vi "Helium Test - Step 1.vi"(7 "Step":i32, 8 "error in":errorcluster, 9 "Test Results In":T9, 10 "Gas":T8, 11 "Test Configuration":T1) -> (0 "error out":errorcluster, 1 "Test Results Out":T9, 2 "Gas Out":T8 caption="Gas", 3 "Test Configuration Out":T1)   [LabVIEW 2015]
uses:
  CAN Communication/PAS/Typedefs/Session Handle.ctl
  CAN Communication/PAS/PAS.lvclass
  Controls/Test Results.ctl
  Controls/Step Result.ctl
  Controls/Test Configuration.ctl
  Controls/Vacuum Test.ctl
  Controls/Test Timing.ctl
  Controls/Vaccum Thresholds.ctl
  Controls/Helium Test.ctl
  Controls/Helium Thresholds.ctl
  Controls/Functional Test.ctl
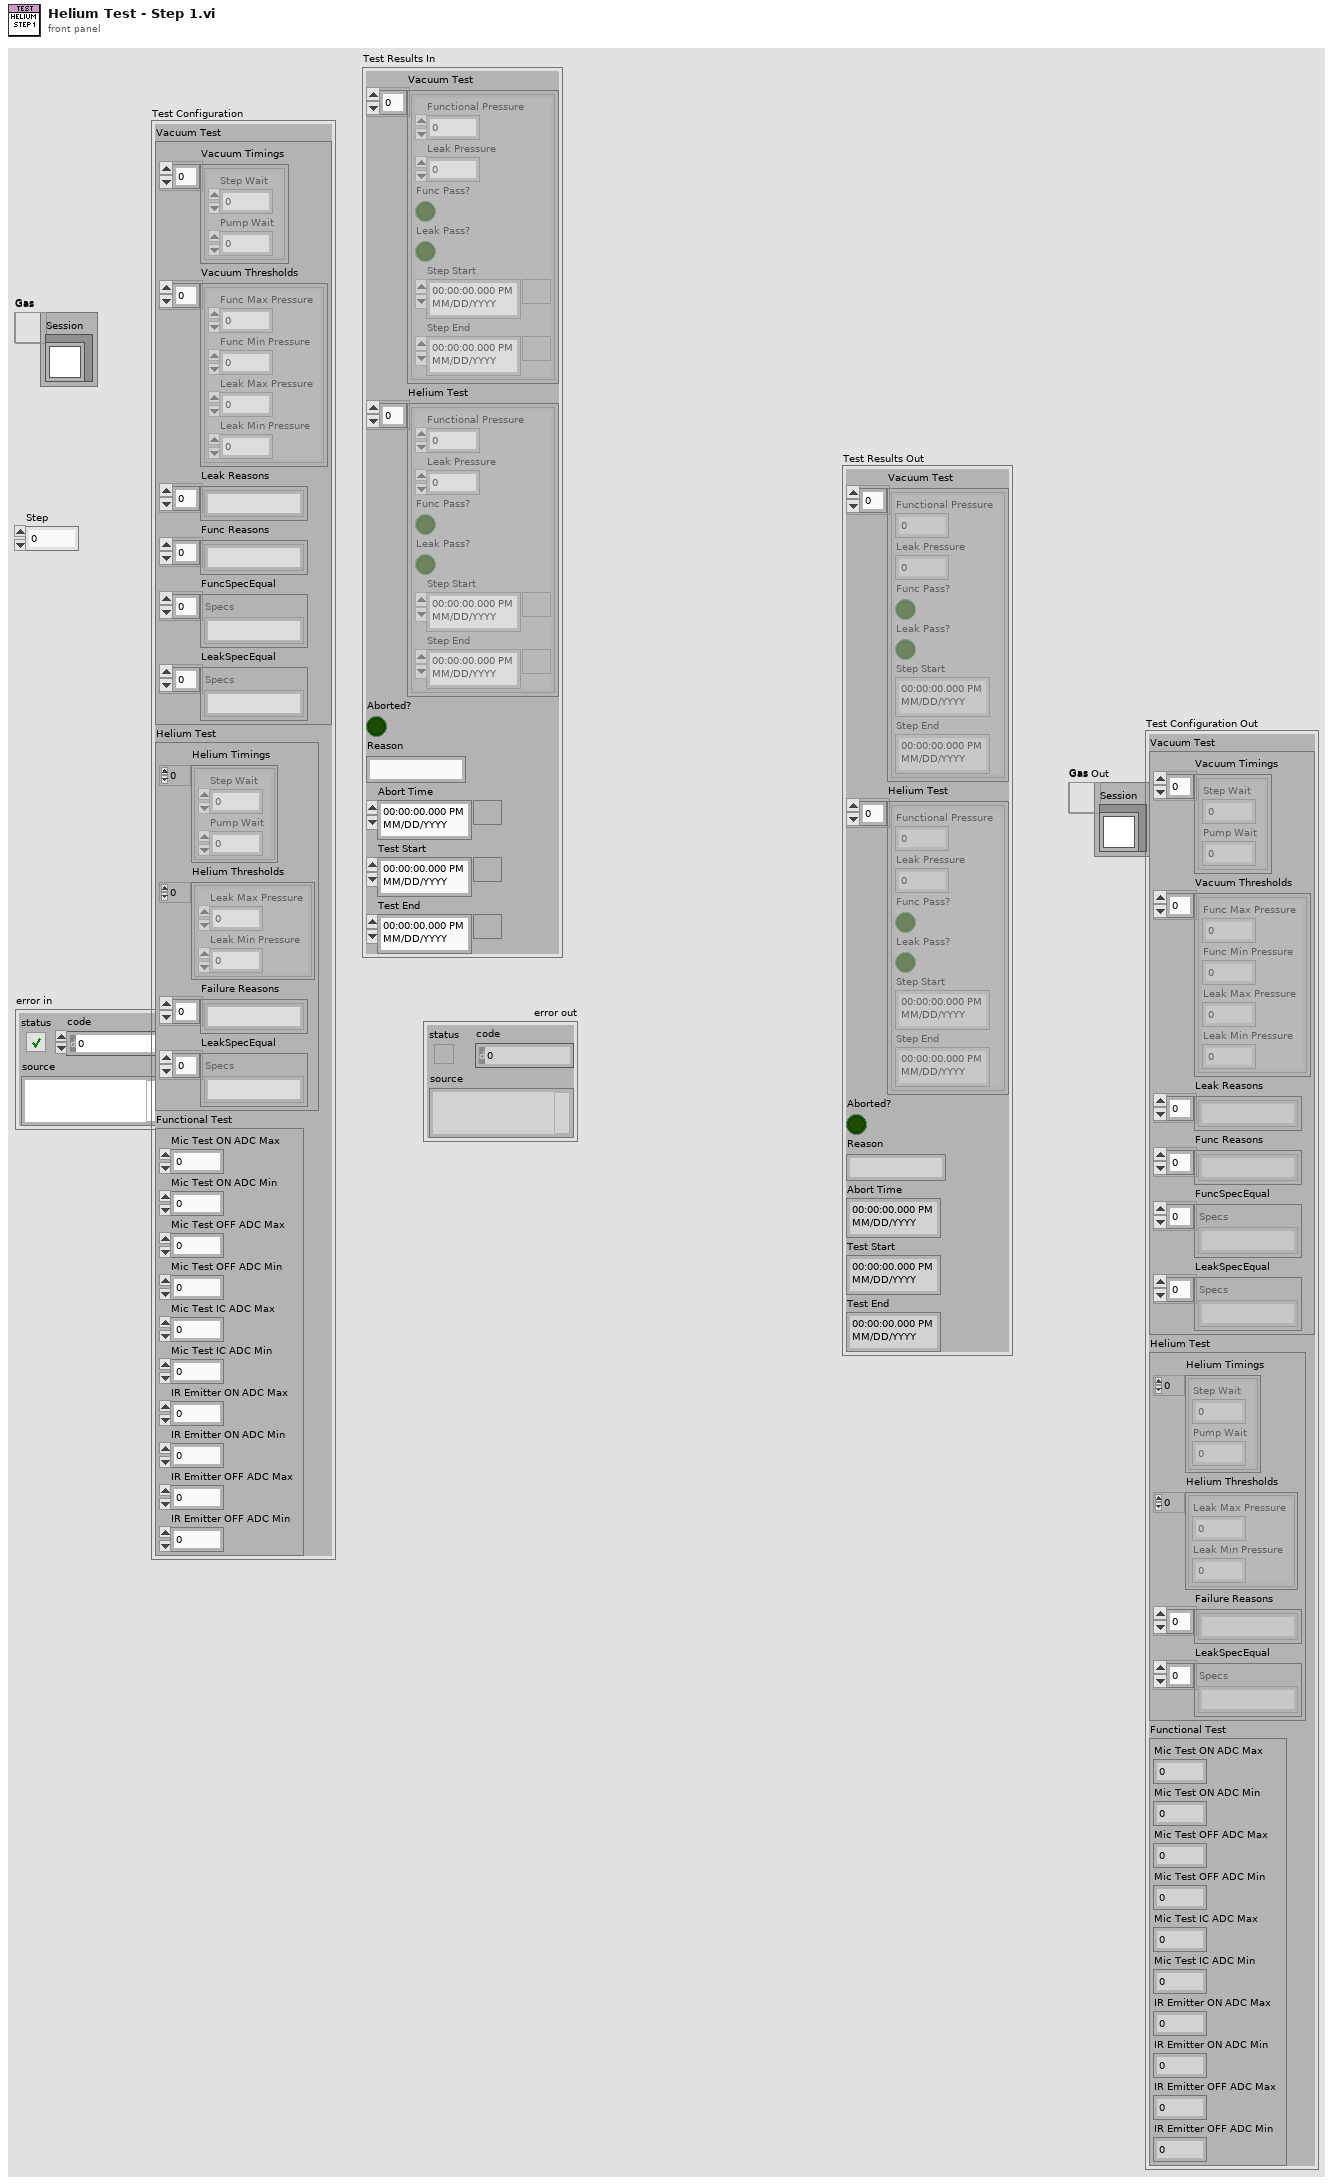
[diagram p1: front panel]
types:
  T1 = typedef "Test Configuration.ctl" = cluster{"Vacuum Test":T2, "Helium Test":T5, "Functional Test":T7}
  T2 = typedef "Vacuum Test.ctl" = cluster{"Vacuum Timings":T3[], "Vacuum Thresholds":T4[], "Leak Reasons":string[], "Func Reasons":string[], "FuncSpecEqual":string[], "LeakSpecEqual":string[]}
  T3 = typedef "Test Timing.ctl" = cluster{"Step Wait":dbl, "Pump Wait":dbl}
  T4 = typedef "Vaccum Thresholds.ctl" = cluster{"Func Max Pressure":dbl, "Func Min Pressure":dbl, "Leak Max Pressure":dbl, "Leak Min Pressure":dbl}
  T5 = typedef "Helium Test.ctl" = cluster{"Helium Timings":T3[], "Helium Thresholds":T6[], "Failure Reasons":string[], "LeakSpecEqual":string[]}
  T6 = typedef "Helium Thresholds.ctl" = cluster{"Leak Max Pressure":dbl, "Leak Min Pressure":dbl}
  T7 = typedef "Functional Test.ctl" = cluster{"Mic Test ON ADC Max":dbl, "Mic Test ON ADC Min":dbl, "Mic Test OFF ADC Max":dbl, "Mic Test OFF ADC Min":dbl, "Mic Test IC ADC Max":dbl, "Mic Test IC ADC Min":dbl, "IR Emitter ON ADC Max":dbl, "IR Emitter ON ADC Min":dbl, "IR Emitter OFF ADC Max":dbl, "IR Emitter OFF ADC Min":dbl}
  T8 = typedef "PAS.lvclass/Session Handle.ctl" = refnum<data-value>
  T9 = typedef "Test Results.ctl" = cluster{"Vacuum Test":T10[], "Helium Test":T10[], "Aborted?":bool, "Reason":string, "Abort Time":timestamp, "Test Start":timestamp, "Test End":timestamp}
  T10 = typedef "Step Result.ctl" = cluster{"Functional Pressure":dbl, "Leak Pressure":dbl, "Func Pass?":bool, "Leak Pass?":bool, "Step Start":timestamp, "Step End":timestamp}
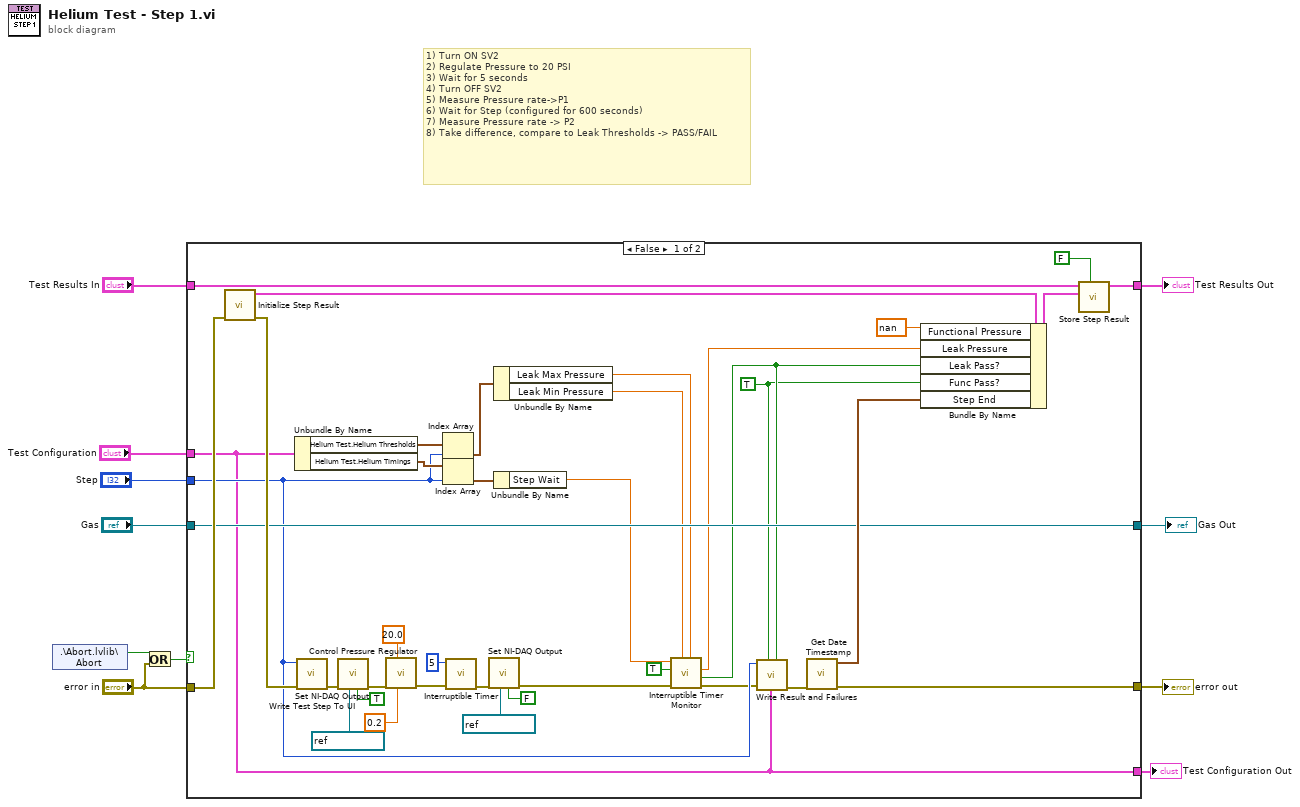
[diagram p0: block diagram]
diagram:
  # "1) Turn ON SV2\n2) Regulate Pressure to 20 PSI\n3) Wait for 5 seconds\n4) Turn OFF SV2\n5) Measure Pressure rate->P1\n6) Wait for Step (configured for 600 seconds)\n7) Measure Pressure rate -> P2\n8) Take difference, compare to Leak Thresholds -> PASS/FAIL"
  n1 = shared-variable ".\\Abort.lvlib\\Abort"() -> (w10:bool)  [unwired: 1 in, 1 out]
  n2 = Or(x=w10, y="error in") -> (x .or. y?=w9:bool)
  n3 = case shown="False" w9 {
    tunnel: "error in" -> [w49 w52]
    tunnel: "Test Results In" -> [w46 w53]
    tunnel: [w47 w53] -> w7
    tunnel: [w12 w52] -> w6
    tunnel: "Test Configuration" -> [w36 w51]
    tunnel: "Step" -> [w37 _]
    tunnel: [w36 w51] -> w1
    tunnel: [w39 w50] -> w3
    tunnel: "Gas" -> [w39 w50]
    frame False {
      w13 = TRUE ("Func Pass?")
      n4 = call "Initialize Step Result.vi"("error in (no error)"=w49) -> ("error out"=w48:errorcluster, "New Step Result"=w45:T10)  [unwired: 8 in, 1 out]
      n5 = Unbundle By Name(w36) -> ("Helium Test.Helium Thresholds"=w42:T6[], "Helium Test.Helium Timings"=w41:T3[])
      n6 = call "Write Test Step To UI.vi"("error in (no error)"=w48, "Step"=w37) -> ("error out"=w27:errorcluster)  [unwired: 9 in]
      n7 = call "Set NI-DAQ Output.vi"("State"=TRUE, "Channel"=refnum<k21> "SV2_PAS", "error in (no error)"=w27) -> ("error out"=w30:errorcluster)  [unwired: 8 in]
      n8 = call "Control Pressure Regulator.vi"("y"=0.2, "error in"=w30, "Desired PSI"=20.0) -> ("error out"=w28:errorcluster)  [unwired: 7 in, 1 out]
      n9 = Index Array(array=w42, index=w37) -> (element=w38:T6)
      n10 = Index Array(array=w41, index=w37) -> (element=w40:T3)
      n11 = call "Interruptible Timer.vi"("error in (no error)"=w28, "Wait (s)"=5) -> ("error out"=w26:errorcluster)  [unwired: 7 in, 2 out]
      n12 = call "Set NI-DAQ Output.vi"("State"=FALSE, "Channel"=refnum<k21> "SV2_PAS", "error in (no error)"=w26) -> ("error out"=w19:errorcluster)  [unwired: 8 in]
      n13 = Unbundle By Name(w38) -> ("Leak Max Pressure"=w21:dbl, "Leak Min Pressure"=w22:dbl)
      n14 = Unbundle By Name(w40) -> ("Step Wait"=w24:dbl)
      n15 = call "Interruptible Timer Monitor.vi"("Max"=w21, "Min"=w22, "error in (no error)"=w19, "Update UI?"=TRUE, "Wait (s)"=w24) -> ("error out"=w15:errorcluster, "In Range?"=w18:bool, "Leak Rate"=w20:dbl)  [unwired: 3 in, 1 out]
      n16 = call "Write Result and Failures.vi"("Leak"=w18, "Test Configuration"=w36, "Func"=w13, "error in (no error)"=w15, "Step"=w37) -> ("error out"=w14:errorcluster)  [unwired: 6 in]
      n17 = call "Get Date Timestamp.vi"("error in (no error)"=w14) -> ("error out"=w12:errorcluster, "current time"=w43:timestamp)  [unwired: 9 in]
      n18 = Bundle By Name(cluster=w45, "Functional Pressure"=nan, "Leak Pressure"=w20, "Leak Pass?"=w18, "Func Pass?"=w13, "Step End"=w43) -> (w44:T10)
      n19 = call "Store Step Result.vi"("Vacuum?"=FALSE, "Step Result"=w44, "Test Results In"=w46) -> ("Test Results Out"=w47:T9)  [unwired: 8 in]
    }
    frame True {
    }
  }
  "error out" <- w6
  "Test Results Out" <- w7
  "Gas Out" <- w3
  "Test Configuration Out" <- w1
